vi "File.Rename Files with Date Modified and Incrementing Number.vi"(8 "Include Date Modified":bool, 9 "Digit Len":i32=3, 10 "New Name":string, 11 "Folder":path) -> (0 "error out":errorcluster, 2 "File Count":i32)   [LabVIEW 2019]
uses:
  <vilib>/KATE/Files/File Utils.lvlib
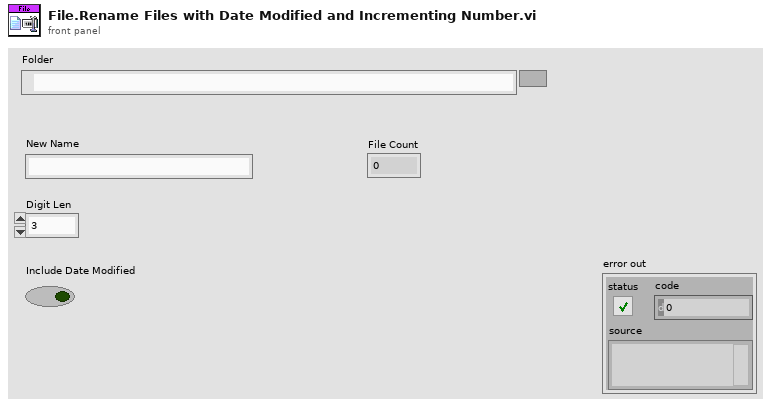
[diagram p1: front panel]
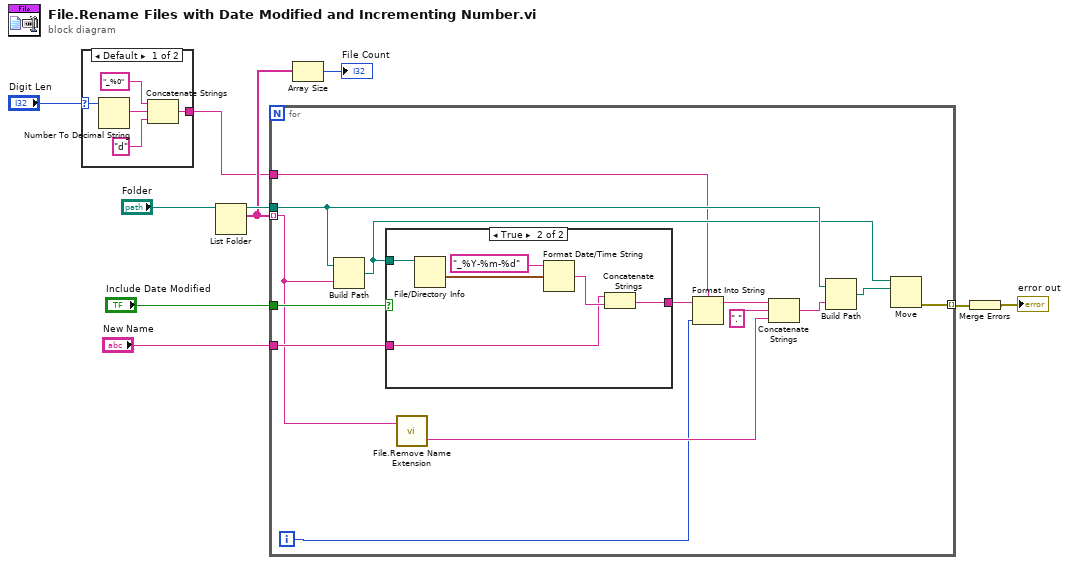
[diagram p0: block diagram]
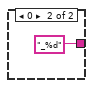
[diagram p2: hidden frame]
diagram:
  n1 = case shown="Default" "Digit Len" {
    selector: "Digit Len" -> [w15 _]
    tunnel: [w11 "_%d" ("format string")] -> w1
    frame Default {
      n2 = Number To Decimal String(number=w15) -> (decimal integer string=w14:string)  [unwired: 1 in]
      n3 = Concatenate Strings("_%0" ("format string"), w14, "d" ("format string")) -> (w11:string)
    }
    frame 0 {
    }
  }
  n4 = List Folder(path="Folder") -> (path out=w9:path, filenames=w6:string[])  [unwired: 3 in, 2 out]
  n5 = for {
    tunnel: w9 -> [w23]
    tunnel: w6 -> [w17] mode=indexing
    tunnel: "New Name" -> [w29]
    tunnel: "Include Date Modified" -> [w30]
    tunnel: [w20] -> w4 mode=indexing
    tunnel: w1 -> [w18]
    i -> [w19]
    n6 = Build Path(base path=w23, name or relative path=w17) -> (appended path=w21:path)
    n7 = case shown="True" w30 {
      tunnel: w29 -> [w31 w34]
      tunnel: [w31 w33] -> w28
      tunnel: w21 -> [_ w32]
      frame False {
      }
      frame True {
        n8 = File/Directory Info(path=w32) -> (last mod=w37:timestamp)  [unwired: 1 in, 6 out]
        n9 = Format Date/Time String(time format string (%c)="_%Y-%m-%d", seconds (now)=w37) -> (date/time string=w35:string)  [unwired: 1 in]
        n10 = Concatenate Strings(w34, w35) -> (w33:string)
      }
    }
    n11 = call <vilib>:"File.Remove Name Extension.vi"("File Name"=w17) -> ("Ext"=w25:string)  [unwired: 1 in, 1 out]
    n12 = Format Into String(format string=w18, initial string=w28, w19) -> (resulting string=w27:string)  [unwired: 1 in, 1 out]
    n13 = Concatenate Strings(w27, "." ("format string"), w25) -> (w24:string)
    n14 = Build Path(base path=w23, name or relative path=w24) -> (appended path=w22:path)
    n15 = Move(source path=w21, 10:w22) -> (error out=w20:errorcluster)  [unwired: 3 in, 2 out]
  }
  n16 = Array Size(array=w6) -> (size(s)=→"File Count":i32)
  n17 = Merge Errors(w4) -> (→"error out":errorcluster)
